vi "test_3_初始化窗口.vi"   [LabVIEW 2012]
uses:
  LabView4Las.dll
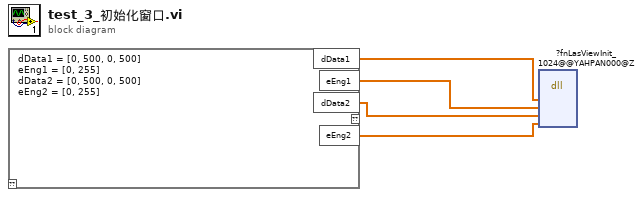
[diagram p0: block diagram]
diagram:
  n1 = script code="dData1 = [0, 500, 0, 500]\neEng1 = [0, 255]\ndData2 = [0, 500, 0, 500]\neEng2 = [0, 255]"() -> ("dData1"=w4:cdb[], "eEng1"=w3:cdb[], "dData2"=w2:cdb[], "eEng2"=w1:cdb[])  [unwired: 1 in, 1 out]
  n2 = dll-call lib="C:/Developer/labview/dll2/LabView4Las.dll" fn="?fnLasViewInit_1024@@YAHPAN000@Z"("dData1"=w4, "eEng1"=w3, "dData2"=w2, "eEng2"=w1) -> ()  [unwired: 8 in, 2 out]
